vi "Tool Q LEIN stroke fb value ovveride MKII with solenoid.vi"(1 "Retry on err (F)":bool, 5 "stroke value(mm)":dbl, 9 "Serial number(any number(-1))":i16=-1, 11 "error in (no error)":errorcluster, 12 "Solenoid override 1":T2, 13 "Solenoid override 2":T2, 14 "Solenoid override 3":T2) -> (15 "error out":errorcluster)   [LabVIEW 2010]
doc: "-1 = any address:\n-2 = do not update"
uses:
  Solenoid overide values.ctl
  solenoid channel override.ctl
  LEINmaster/Defenitions/LEIN Structure variations.ctl
  Application Structure/Options/Action GFV Settings.ctl
panel:
  out "data string":string
  out "Valve 3":u8 format="%08b"
  out "valve 1 and 2":u8 format="%08b"
  in  "Solenoid channel overide":T1
  # "-1 = any address:\n-2 =  do not update"
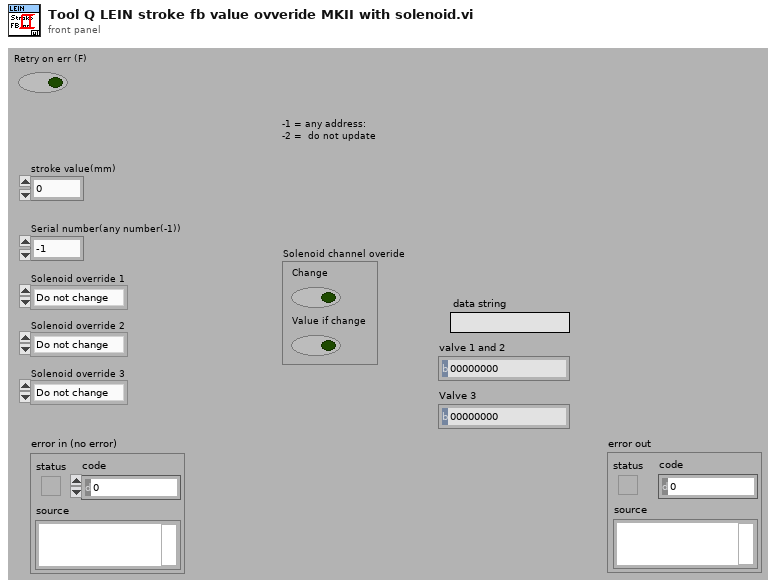
[diagram p1: front panel]
types:
  T1 = typedef "solenoid channel override.ctl" = cluster{"Change":bool, "Value if change":bool}
  T2 = typedef "Solenoid overide values.ctl" = enum16{"Do not change", "Open", "Close", "NA (0-0)", "NA (1-1)"}
  T3 = enum16{"big-endian, network order", "native, host order", "little-endian"}
  T4 = typedef "Action GFV Settings.ctl" = enum16{"Init", "Get From INI", "Put In INI", "Get Settings", "Get Update Index", "Set Setting"}
  T5 = typedef "LEIN Structure variations.ctl" = enum16{"LEIN08", "LEIN31", "LEIN63"}
  T6 = typedef "Options  All pages and custom.ctl" = cluster{"P 1 (App)":T7, "P 2":T8, "P 3":T9, "P 4":T11, "P 5":T14, "P 6 (Err)":T15, "P 7 (Expert)":T16, "C 1":T18, "C 2":T19}
  T7 = typedef "Options Page 1 (App).ctl" = cluster{"Result files":path, "PCP Interface":string, "Modem Interface":string}
  T8 = typedef "Options Page 2.ctl" = cluster{"Audible Alarm":bool, "Force alarm on Technical":bool, "Force alarm on HH":bool, "Force alarm on LL":bool, "Force alarm on H":bool, "Force alarm on L":bool}
  T9 = typedef "Options Page 3.ctl" = cluster{"Min resistance":dbl, "Max resistance":dbl, "PCP/PSU range":T10, "Max voltage jump":dbl, "Maximum resistance change":dbl}
  T10 = typedef "PCP type List.ctl" = enum16{"0 - 350V", "0 - 450V", "0 - 600V"}
  T11 = typedef "Options Page 4.ctl" = cluster{"relay 1":dbl, "Relay 2":dbl, "Solenoid limit":dbl, "Force det.":T12, "Stroke force lim.":dbl, "Pressure SLIPS":dbl, "Tacometer puls":dbl, "Stroke force":T13}
  T12 = typedef "Stroke force selector.ctl" = enum16{"Stroke in = node 1", "Strok out = node 1"}
  T13 = typedef "Stroke force calculation.ctl" = enum16{"Node 1 minus Node 2", "Node 2 minus Node 1"}
  T14 = typedef "Options Page 5.ctl" = cluster{"Placeholder":bool}
  T15 = typedef "Options Page 6 (Err).ctl" = cluster{"Error and event files":path}
  T16 = typedef "Options Page 7 (Expert).ctl" = cluster{"Show Debug":bool, "Log debug messages":bool, "Aditional debug messages":bool, "enumCANCOM":bool, "AutoLogOn":bool, "Buffer size":i32, "Modem sim":T17, "Modem baud":u16, "Upd regular data":bool}
  T17 = typedef "Modem simulation setup.ctl" = cluster{"Modem dealay sim":bool, "Sim baud Tx":u16, "Bit Error fraction Tx":dbl, "Sim baud Rx":u16, "Bit Error fraction Rx":dbl}
  T18 = typedef "Options Custom 1.ctl" = cluster{"Placeholder":bool}
  T19 = typedef "Options Custom 2.ctl" = cluster{"Placeholder":bool}
  T20 = typedef "LEIN CMD Cluster.ctl" = cluster{"SID":u8, "ANF":bool, "CMD":T21, "DATA":u8[]}
  T21 = typedef "LEIN CMD List.ctl" = enum8{"ACTI", "TASK", "RES0", "STAT", "RES1", "RES2", "RES3", "USER"}
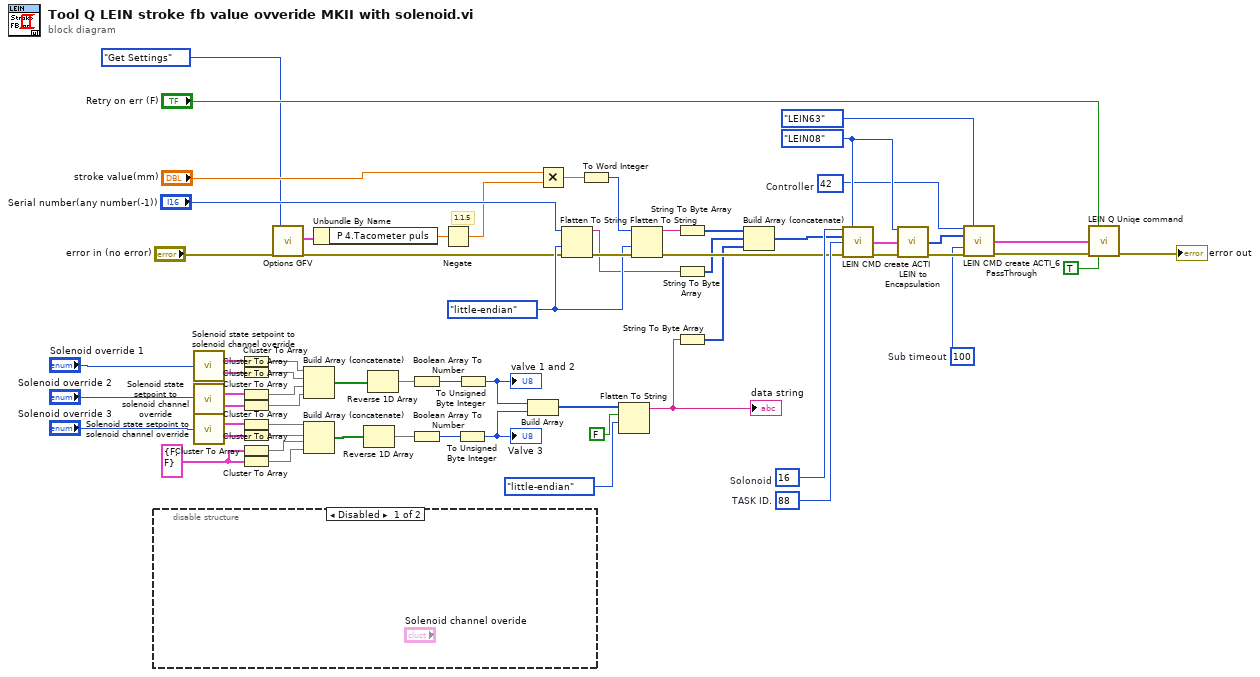
[diagram p0: block diagram]
diagram:
  w5 = T1 {"Change"=FALSE, "Value if change"=FALSE} ("Close")
  w47 = u8 42  # Controller
  w48 = u8 16  # Solonoid
  w54 = u16 100  # Sub timeout
  w51 = u8 88  # TASK ID.
  w50 = LEIN_Structure_variations."LEIN08" ("LEIN Variation")
  w41 = T3."little-endian" ("byte order (0:big-endian, network order)")
  # "1.1.5"
  n1 = disable-structure shown="Disabled" {
    frame Disabled {
    }
    frame Enabled {
    }
  }
  n2 = call "Solenoid state setpoint to solenoid channel override.vi"("Solenoid override 1"="Solenoid override 1") -> ("Open"=w28:T1, "Close"=w27:T1)  [unwired: 13 in]
  n3 = call "Solenoid state setpoint to solenoid channel override.vi"("Solenoid override 1"="Solenoid override 2") -> ("Open"=w26:T1, "Close"=w25:T1)  [unwired: 13 in]
  n4 = call "Solenoid state setpoint to solenoid channel override.vi"("Solenoid override 1"="Solenoid override 3") -> ("Open"=w24:T1, "Close"=w23:T1)  [unwired: 13 in]
  n5 = Cluster To Array(cluster=w28) -> (array=w22:bool[])
  n6 = Cluster To Array(cluster=w27) -> (array=w21:bool[])
  n7 = Cluster To Array(cluster=w26) -> (array=w20:bool[])
  n8 = Cluster To Array(cluster=w25) -> (array=w19:bool[])
  n9 = Cluster To Array(cluster=w24) -> (array=w16:bool[])
  n10 = Cluster To Array(cluster=w23) -> (array=w15:bool[])
  n11 = Cluster To Array(cluster=w5) -> (array=w4:bool[])
  n12 = Cluster To Array(cluster=w5) -> (array=w3:bool[])
  n13 = call "Options GFV.vi"("error in (no error)"="error in (no error)", "Action(Get Settings)"=Action_GFV_Settings."Get Settings") -> ("Options"=w34:T6, "error out"=w35:errorcluster)  [unwired: 15 in, 1 out]
  n14 = Build Array (concatenate)(w22, w21, w20, w19) -> (w18:bool[])
  n15 = Build Array (concatenate)(w16, w15, w4, w3) -> (w17:bool[])
  n16 = Unbundle By Name(w34) -> ("P 4.Tacometer puls"=w33:dbl)
  n17 = Reverse 1D Array(array=w17) -> (reversed array=w11:bool[])
  n18 = Reverse 1D Array(array=w18) -> (reversed array=w12:bool[])
  n19 = Boolean Array To Number(Boolean array=w12) -> (number=w14:u32)
  n20 = Boolean Array To Number(Boolean array=w11) -> (number=w13:u32)
  n21 = Negate(x=w33) -> (-x=w32:dbl)
  n22 = To Unsigned Byte Integer(number=w13) -> (unsigned 8bit integer=w9:u8)
  "Valve 3" <- w9
  n23 = To Unsigned Byte Integer(number=w14) -> (unsigned 8bit integer=w10:u8)
  "valve 1 and 2" <- w10
  n24 = Build Array(w10, w9) -> (w7:u8[])
  n25 = Multiply(x="stroke value(mm)", y=w32) -> (x*y=w63:dbl)
  n26 = Flatten To String(anything="Serial number(any number(-1))", byte order (0:big-endian, network order)=w41, error in (no error)=w35) -> (data string=w39:string, error out=w42:errorcluster)  [unwired: 1 in, 1 out]
  n27 = To Word Integer(number=w63) -> (16bit integer=w62:i16)
  n28 = Flatten To String(anything=w7, prepend array or string size? (T)=FALSE, byte order (0:big-endian, network order)=T3."little-endian") -> (data string=w2:string)  [unwired: 1 in, 2 out]
  "data string" <- w2
  n29 = Flatten To String(anything=w62, byte order (0:big-endian, network order)=w41, error in (no error)=w42) -> (data string=w61:string, error out=w44:errorcluster)  [unwired: 1 in, 1 out]
  n30 = String To Byte Array(string=w61) -> (unsigned byte array=w49:u8[])
  n31 = String To Byte Array(string=w39) -> (unsigned byte array=w38:u8[])
  n32 = String To Byte Array(string=w2) -> (unsigned byte array=w1:u8[])
  n33 = Build Array (concatenate)(w49, w38, w1) -> (w43:u8[])
  n34 = call "LEIN CMD create ACTI.vi"("SID"=w48, "LEIN Variation"=w50, "Data"=w43, "ACTI ID"=w51, "error in (no error)"=w44) -> ("CMD"=w52:T20, "error out"=w53:errorcluster)  [unwired: 9 in]
  n35 = call "LEIN to Encapsulation.vi"("LEIN Variation"=w50, "CMD"=w52, "error in (no error)"=w53) -> ("Data and header"=w57:u8[], "error out"=w58:errorcluster)  [unwired: 8 in, 3 out]
  n36 = call "LEIN CMD create ACTI_6 PassThrough.vi"("SID"=w47, "LEIN Variation"=LEIN_Structure_variations."LEIN63", "LEIN ecapsulated data (header and data)"=w57, "Sub Timeout (ms)"=w54, "error in (no error)"=w58) -> ("CMD"=w56:T20, "error out"=w55:errorcluster)  [unwired: 9 in]
  n37 = call "LEIN Q Uniqe command.vi"("Retry on err (F)"="Retry on err (F)", "CMD"=w56, "error in"=w55, "priority(F)"=TRUE) -> ("error out"=→"error out":errorcluster)  [unwired: 11 in]
